vi "Process Sample Set.vi"(8 "error in (no error)":errorcluster, 11 "Sample Set in":dbl[](array[numeric])) -> (0 "error out":errorcluster, 2 "Valid?":bool, 3 "Sample Set out":dbl[](array[numeric]))   [LabVIEW 2011]
uses:
  <vilib>/Analysis/NI_AALBase.lvlib
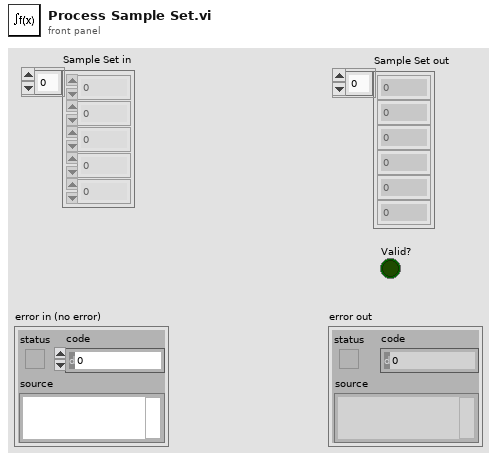
[diagram p1: front panel]
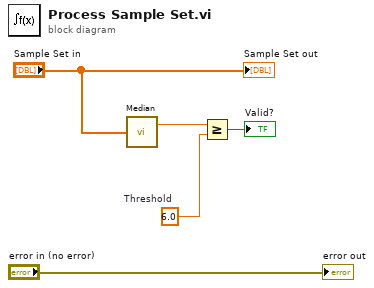
[diagram p0: block diagram]
diagram:
  w3 = 6.0  # Threshold
  n1 = call <vilib>:"Median.vi"("X"="Sample Set in") -> ("median"=w4:dbl)  [unwired: 1 out]
  n2 = Greater Or Equal?(x=w4, y=w3) -> (x >= y?=→"Valid?":bool)
  "error out" <- "error in (no error)"
  "Sample Set out" <- "Sample Set in"
